vi "_TangoDeviceCommandsList.vi"(0 "device name":string) -> (2 "commands_list":string[](array[string]))   [LabVIEW 2014, in "tango.lvlib"]
uses:
  tango.lvlib
  tango_binding.dll
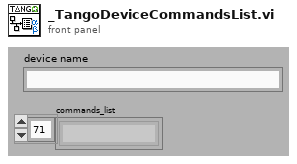
[diagram p1: front panel]
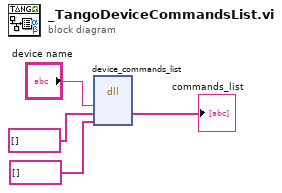
[diagram p0: block diagram]
diagram:
  n1 = dll-call lib="tango_binding.*" fn="device_commands_list"("dev_name"="device name", "attributes_list"=string[] [] ("Error Stack"), "error_stack"=string[] [] ("Error Stack")) -> ("attributes_list"=→"commands_list":string[])  [unwired: 6 in, 2 out]
